vi "get_stage_loc.vi"(11 "error in (no error)":errorcluster) -> (3 "String":string)   [LabVIEW 2016]
uses:
  <vilib>/Instr/_visa.llb/VISA Configure Serial Port (Instr).vi
panel:
  out "error out":errorcluster
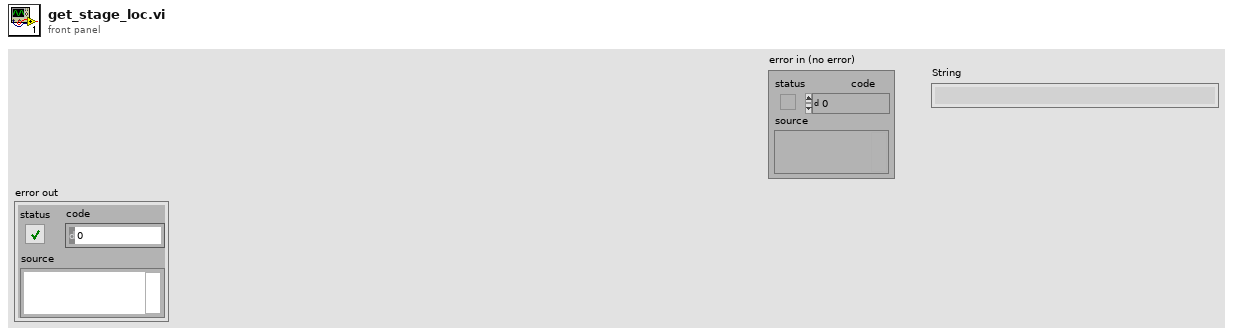
[diagram p1: front panel]
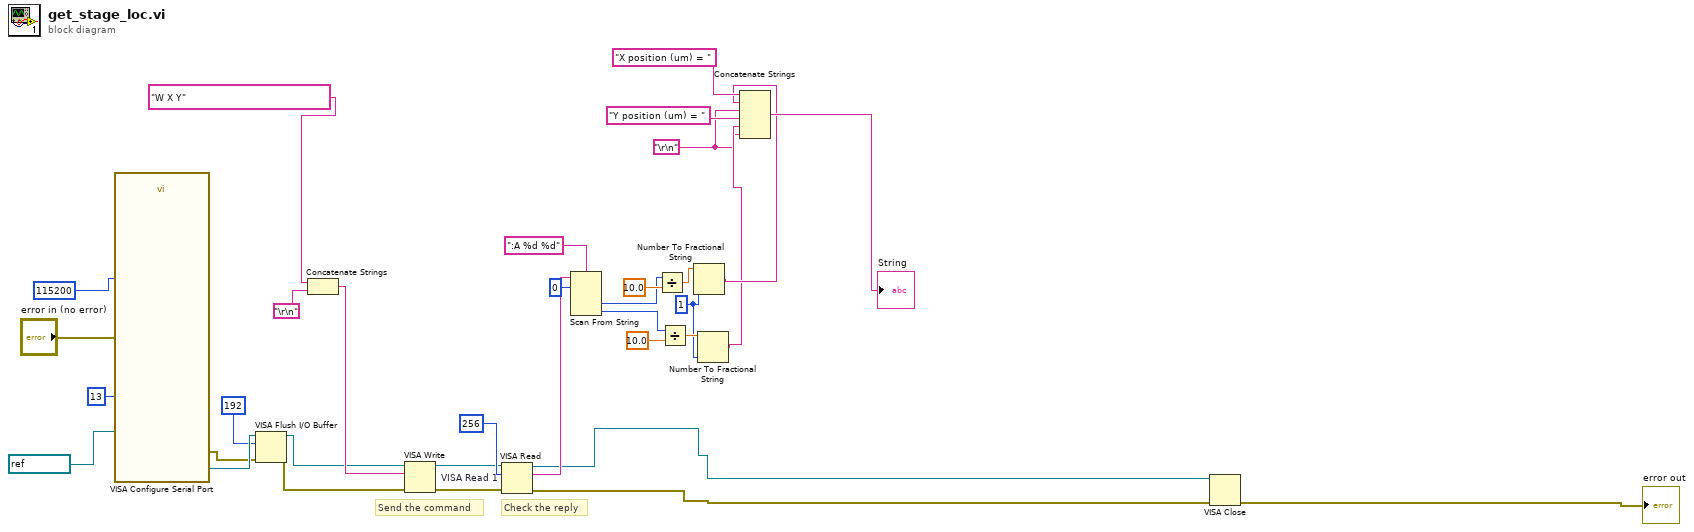
[diagram p0: block diagram]
diagram:
  w1 = "\r\n"
  w5 = i16 1 ("precision (6)")
  # "Check the reply"
  # "Send the command"
  n1 = call-poly "VISA Configure Serial Port"("VISA resource name"=refnum<visa-resource-name> "COM6", "termination char\n(0xA = '\\n' = LF)"=u8 13 ("termination char\n(0xA = '\\n' = LF)"), "baud rate (9600)"=u32 115200, "error in (no error)"="error in (no error)") -> ("VISA resource name out"=w24:refnum<visa-resource-name>, "error out"=w23:errorcluster)  [unwired: 3 in, 7 out]
  n2 = VISA Flush I/O Buffer(VISA resource name=w24, mask (16)=u16 192 ("Mask"), error in (no error)=w23) -> (VISA resource name out=w21:refnum<visa-resource-name>, error out=w20:errorcluster)
  n3 = Concatenate Strings("W X Y" ("write buffer"), "\r\n") -> (w29:string)
  n4 = VISA Write(VISA resource name=w21, write buffer=w29, error in (no error)=w20) -> (VISA resource name out=w18:refnum<visa-resource-name>, error out=w17:errorcluster)  [unwired: 1 out]
  n5 = VISA Read "VISA Read 1"(VISA resource name=w18, byte count=u32 256, error in (no error)=w17) -> (VISA resource name out=w16:refnum<visa-resource-name>, read buffer=w31:string, error out=w15:errorcluster)  [unwired: 1 out]
  n6 = Scan From String(format string=":A %d %d", input string=w31, initial scan location=u32 0) -> (output 1=w12:i32, output 2=w10:i32)  [unwired: 3 in, 3 out]
  n7 = Divide(x=w12, y=10.0) -> (x/y=w8:dbl)
  n8 = Divide(x=w10, y=10.0) -> (x/y=w6:dbl)
  n9 = Number To Fractional String(number=w8, precision (6)=w5) -> (F-format string=w7:string)  [unwired: 2 in]
  n10 = Number To Fractional String(number=w6, precision (6)=w5) -> (F-format string=w3:string)  [unwired: 2 in]
  n11 = Concatenate Strings("X position (um) = " ("string"), w7, w1, "Y position (um) = " ("string"), w3, w1) -> (→"String":string)
  n12 = VISA Close(VISA resource name=w16, error in (no error)=w15) -> (error out=→"error out":errorcluster)
